vi "Get Node Wild (Usage Mask).vi"(8 "error in (no error)":errorcluster, 9 "Usage mask":i32, 10 "Path":string, 11 "Tree in":refnum<class "Tree.lvclass">) -> (0 "error out":errorcluster, 2 "Node array out":refnum<class "TreeNodeArray.lvclass">, 3 "Tree out":refnum<class "Tree.lvclass">)   [LabVIEW 2015, in "MDSplus.lvlib" / "Tree.lvclass"]
doc: "Return the TreeNode array for all the successor nodes of the specified usage with respect of the passed path."
uses:
  Tree.lvclass
  TreeNodeArray_Class/TreeNodeArray.lvclass
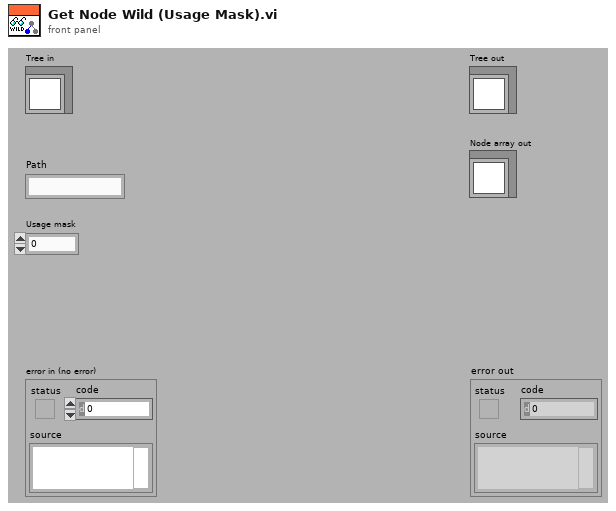
[diagram p1: front panel]
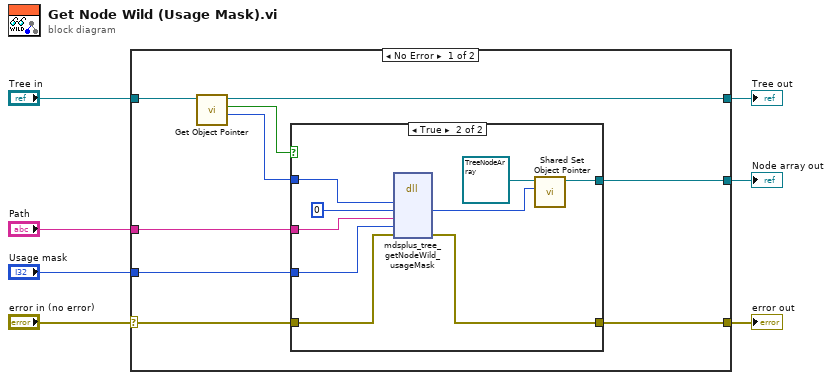
[diagram p0: block diagram]
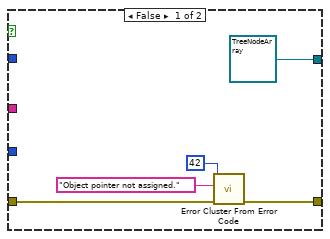
[diagram p2: hidden frame]
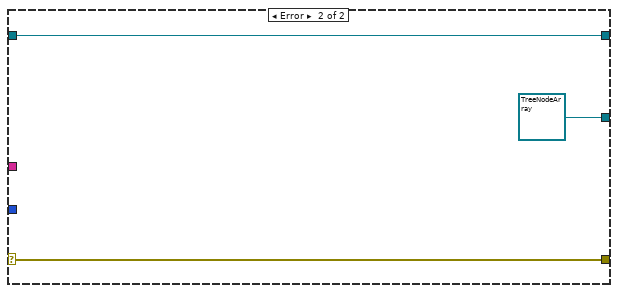
[diagram p3: hidden frame]
diagram:
  n1 = case shown="No Error" "error in (no error)" {
    selector: "error in (no error)" -> [w10 w33]
    tunnel: [w9 w33] -> w6
    tunnel: [w15 w32] -> w4
    tunnel: "Tree in" -> [w16 w32]
    tunnel: "Path" -> [w14 _]
    tunnel: [w13 refnum<class "TreeNodeArray.lvclass"> refnum ("TreeNode out")] -> w2
    tunnel: "Usage mask" -> [w8 _]
    frame No Error {
      n2 = call-dynamic "Get Object Pointer.vi"("Tree in"=w16) -> ("Object Pointer"=w11:i64, "Assigned object pointer?"=w12:bool, "Tree out"=w15:refnum<class "Tree.lvclass">)  [unwired: 8 in]
      n3 = case shown="True" w12 {
        tunnel: w14 -> [_ w29]
        tunnel: [refnum<class "TreeNodeArray.lvclass"> refnum ("Data out") w26] -> w13
        tunnel: w11 -> [_ w25]
        tunnel: w10 -> [w18 w24]
        tunnel: [w17 w23] -> w9
        tunnel: w8 -> [_ w22]
        frame False {
          n4 = call <vilib>:"Error Cluster From Error Code.vi"("error in (no error)"=w18, "error message (\"\")"="Object pointer not assigned." ("error message (\"\")"), "error code (0)"=42) -> ("error out"=w17:errorcluster)  [unwired: 6 in]
        }
        frame True {
          n5 = dll-call lib="MDSobjectsLVShr" fn="mdsplus_tree_getNodeWild_usageMask"("lvTreePtr"=w25, "lvTreeNodeArrayPtrOut"=i64 0 ("lvTreeNodePtr"), "pathIn"=w29, "usageMaskIn"=w22, "error"=w24) -> ("lvTreeNodeArrayPtrOut"=w27:i64, "error"=w23:errorcluster)  [unwired: 7 in, 2 out]
          n6 = call "Shared Set Object Pointer.vi"("Object Pointer"=w27, "TreeNodeArray in"=refnum<class "TreeNodeArray.lvclass"> refnum ("TreeNode")) -> ("TreeNodeArray out"=w26:refnum<class "TreeNodeArray.lvclass">)  [unwired: 9 in]
        }
      }
    }
    frame Error {
    }
  }
  "error out" <- w6
  "Tree out" <- w4
  "Node array out" <- w2
